vi "test_libssh2_channel_wait_closed.vi"() -> ()   [LabVIEW 2013, in "libssh2_integration_tests.lvlib"]
uses:
  libssh2_integration_tests.lvlib
  <vilib>/addons/_JKI Toolkits/Caraya/classes/Test/Test.lvclass
  support/support.lvlib
  libssh2/libssh2.lvlib
  <vilib>/addons/_JKI Toolkits/Caraya/classes/Assert/Assert.lvclass
panel:
  out "error out":errorcluster
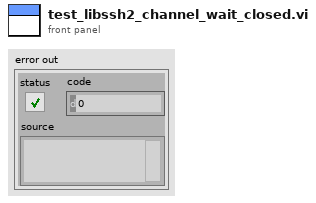
[diagram p1: front panel]
types:
  T1 = typedef "libssh2.lvlib/Session Refnum.ctl" = refnum<k1>
  T2 = typedef "libssh2.lvlib/Channel Refnum.ctl" = refnum<k1>
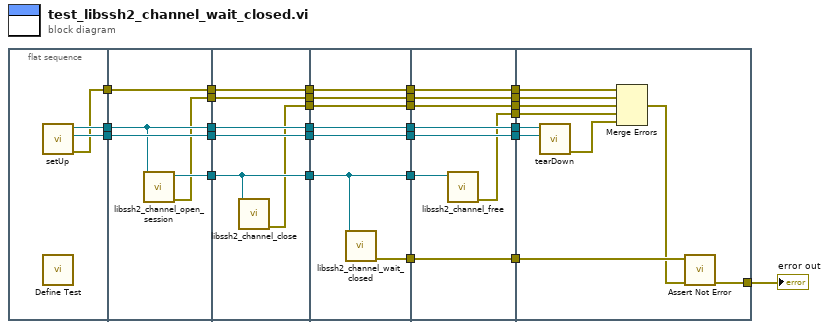
[diagram p0: block diagram]
diagram:
  n1 = flat-sequence {
    tunnel: [w32] -> w29
    tunnel: [w31] -> w28
    tunnel: [w30] -> w18
    tunnel: w29 -> [w36]
    tunnel: w28 -> [w37]
    tunnel: [w36] -> w27
    tunnel: [w37] -> w26
    tunnel: [w35] -> w25
    tunnel: w18 -> [w34]
    tunnel: [w34] -> w17
    tunnel: [w33] -> w15
    tunnel: w27 -> [w43]
    tunnel: w26 -> [w42]
    tunnel: w25 -> [w41]
    tunnel: [w43] -> w13
    tunnel: [w42] -> w11
    tunnel: [w41] -> w9
    tunnel: w17 -> [w40]
    tunnel: [w40] -> w7
    tunnel: w15 -> [w39]
    tunnel: [w39] -> w4
    tunnel: [w38] -> w2
    tunnel: w13 -> [w50]
    tunnel: [w50] -> w12
    tunnel: w11 -> [w49]
    tunnel: [w49] -> w10
    tunnel: w9 -> [w45]
    tunnel: [w45] -> w8
    tunnel: w7 -> [w48]
    tunnel: [w48] -> w6
    tunnel: [w44] -> w5
    tunnel: w4 -> [w47]
    tunnel: [w47] -> w3
    tunnel: w2 -> [w46]
    tunnel: [w46] -> w1
    tunnel: w12 -> [w58]
    tunnel: w10 -> [w57]
    tunnel: w8 -> [w55]
    tunnel: [w58] -> w24
    tunnel: [w57] -> w23
    tunnel: [w56] -> w22
    tunnel: [w54] -> w20
    tunnel: [w53] -> w19
    tunnel: w6 -> [w52]
    tunnel: [w52] -> w16
    tunnel: w5 -> [w56]
    tunnel: w3 -> [w53]
    tunnel: w1 -> [w51]
    tunnel: [w51] -> w14
    tunnel: w24 -> [w67]
    tunnel: w23 -> [w66]
    tunnel: w22 -> [w68]
    tunnel: [w65] -> w21
    tunnel: w20 -> [w63]
    tunnel: w19 -> [w62]
    tunnel: w16 -> [w61]
    tunnel: w14 -> [w59]
    frame #0 {
      n2 = call "setUp.vi"() -> ("error out"=w30:errorcluster, "connection ID"=w31:refnum<k5>, "session"=w32:T1)  [unwired: 9 in]
      n3 = call <vilib>:"Define Test.vi"() -> ()  [unwired: 10 in, 2 out]
    }
    frame #1 {
      n4 = call "libssh2_channel_open_session.vi"("session"=w36) -> ("error out"=w33:errorcluster, "channel"=w35:T2)  [unwired: 9 in]
    }
    frame #2 {
      n5 = call "libssh2_channel_close.vi"("channel"=w41) -> ("error out"=w38:errorcluster)  [unwired: 10 in]
    }
    frame #3 {
      n6 = call "libssh2_channel_wait_closed.vi"("channel"=w45) -> ("error out"=w44:errorcluster)  [unwired: 10 in]
    }
    frame #4 {
      n7 = call "libssh2_channel_free.vi"("channel"=w55) -> ("error out"=w54:errorcluster)  [unwired: 10 in]
    }
    frame #5 {
      n8 = call "tearDown.vi"("connection ID"=w66, "session"=w67) -> ("error out"=w64:errorcluster)  [unwired: 9 in]
      n9 = Merge Errors(w61, w62, w59, w63, w64) -> (w60:errorcluster)
      n10 = call <vilib>:"Assert Not Error.vi"("error in (no error)"=w60, "Not Error?"=w68) -> ("error out"=w65:errorcluster)  [unwired: 8 in, 1 out]
    }
  }
  "error out" <- w21
